vi "Uninit.vi"(2 "Container State":T1 caption="容器状态", 3 "Display State":T2={"method"=enum."None", "current color"=1, "available black position"=[], "available white position"=[], "Interactive Action"=refnum, "row"=0, "column"=0} caption="显示状态") -> ()   [LabVIEW 2018, in "Othello.xctl"]
doc: "本VI是为《我和LabVIEW》一书编写的示例。\n关于本书的介绍请参考网页：\nhttp://ruanqizhen.spaces.live.com/blog/cns!5852D4F797C53FB6!4310.entry"
uses:
  Othello.xctl
  <vilib>/_xctls/Container State.ctl
  <vilib>/_xctls/XControlSupport.lvlib
  Control/Method Call.ctl
  Control/Pict Ring Chess.ctl
  State.ctl
  Control/Interactive Action.ctl
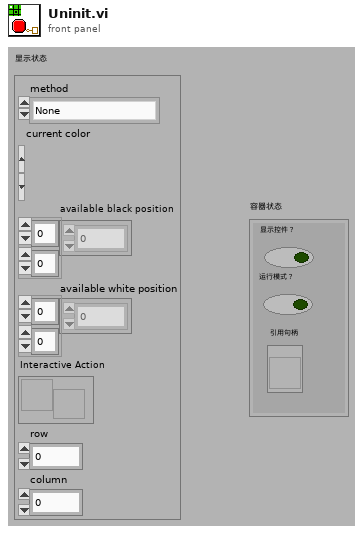
[diagram p1: front panel]
types:
  T1 = typedef "XControlSupport.lvlib/Container State.ctl" = cluster{"Indicator?":bool, "Run Mode?":bool, " Refnum":refnum<vi>}
  T2 = typedef "Othello.xctl/State.ctl" = cluster{"method":T3, "current color":T4, "available black position":i32[][], "available white position":i32[][], "Interactive Action":T5, "row":i32, "column":i32}
  T3 = typedef "Othello.xctl/Method Call.ctl" = enum16{"None", "New Game", "Play One"}
  T4 = typedef "Othello.xctl/Pict Ring Chess.ctl" = u16
  T5 = typedef "Othello.xctl/Interactive Action.ctl" = refnum<user-event>
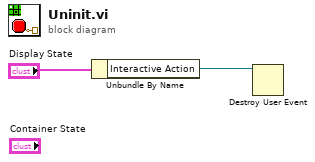
[diagram p0: block diagram]
diagram:
  n1 = Unbundle By Name("Display State") -> ("Interactive Action"=w1:T5)
  n2 = Destroy User Event(user event=w1) -> ()  [unwired: 1 in, 1 out]
